vi "Log Time to File.vi"   [LabVIEW 2011]
doc: "This VI is a daemon that is spawned by the launcher. The delay in the VI allows the laucher time to complete running and return to the idle state. If references are not handled correctly, the launcher will terminate the execution of Hello World before the delay is complete, subsequently the file will not be written. As such, even when references are handled correctly, because of the delay, it will take a moment before the file is written. It is written in the same directory that contains the launcher and the daemon.\n\nAAL 9/09"
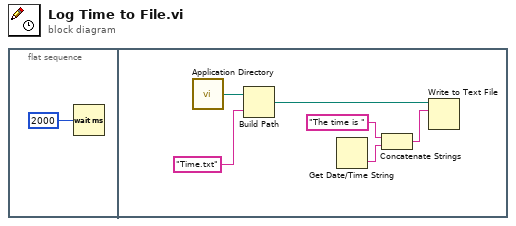
[diagram p0: block diagram]
diagram:
  n1 = flat-sequence {
    frame #0 {
      n2 = Wait (ms)(milliseconds to wait=u32 2000) -> ()  [unwired: 1 out]
    }
    frame #1 {
      n3 = call <vilib>:"Application Directory.vi"() -> ("Application Directory"=w2:path)
      n4 = Build Path(base path=w2, name or relative path="Time.txt") -> (appended path=w4:path)
      n5 = Get Date/Time String() -> (time string=w6:string)  [unwired: 4 out]
      n6 = Concatenate Strings("The time is " ("text"), w6) -> (w5:string)
      n7 = Write to Text File(file (use dialog)=w4, text=w5) -> ()  [unwired: 1 in, 4 out]
    }
  }
